vi "Read AppRef.vi"(8 "error in (no error)":errorcluster, 11 "App Control API in":refnum<class "AppControlAPI.lvclass">) -> (0 "error out":errorcluster, 2 "AppRef":refnum<vi>, 3 "App Control API out":refnum<class "AppControlAPI.lvclass">)   [LabVIEW 2018, in "AppControlAPI.lvclass"]
uses:
  AppControlAPI.lvclass
  AppControlAPI.lvclass/AppControlAPI.ctl
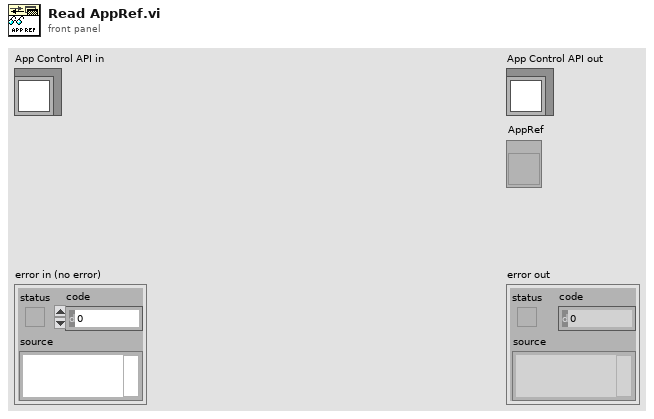
[diagram p1: front panel]
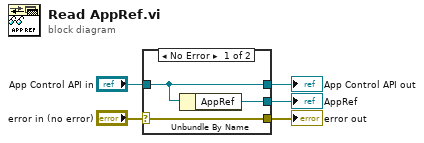
[diagram p0: block diagram]
diagram:
  n1 = case shown="No Error" "error in (no error)" {
    selector: "error in (no error)" -> [w8 w9]
    tunnel: [w8 w9] -> w4
    tunnel: [w7 w10] -> w2
    tunnel: "App Control API in" -> [w7 w10]
    tunnel: [w6 _] -> w1
    frame No Error {
      n2 = Unbundle By Name(w7) -> ("AppRef"=w6:refnum<vi>)
    }
    frame Error {
    }
  }
  "error out" <- w4
  "App Control API out" <- w2
  "AppRef" <- w1
